vi "HW_Gantner_Refresh Tree Device Info.vi"(7 "Cfg":T1[](array[typedef]), 8 "error in":errorcluster caption="错误输入", 10 "Device":string="Device", 11 "Ref.Tree Ref":refnum<vi>) -> (0 "error out":errorcluster caption="错误输出")   [LabVIEW 2016]
uses:
  Ctrls/HardWare _ Module Configuration.ctl
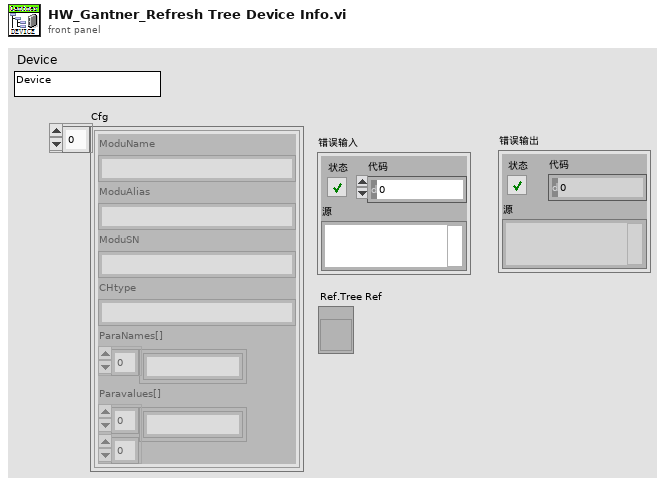
[diagram p1: front panel]
types:
  T1 = typedef "HardWare _ Module Configuration.ctl" = cluster{"ModuName":string, "ModuAlias":string, "ModuSN":string, "CHtype":string, "ParaNames[]":string[], "Paravalues[]":string[][]}
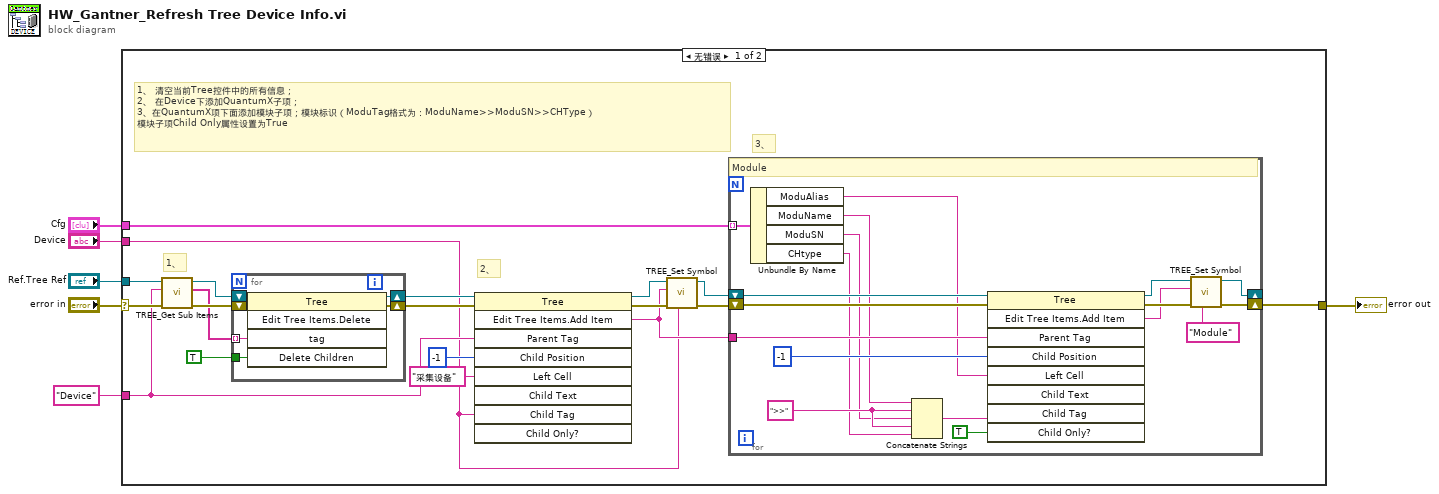
[diagram p0: block diagram]
diagram:
  n1 = case shown="无错误" "error in" {
    selector: "error in" -> [w21 w50]
    tunnel: [w25 w50] -> w5
    tunnel: "Ref.Tree Ref" -> [w19 _]
    tunnel: "Device" ("PicName") -> [w18 _]
    tunnel: "Cfg" -> [w9 _]
    tunnel: "Device" -> [w8 _]
    frame No Error {
      # "3、"
      # "2、"
      # "1、"
      # "1、 清空当前Tree控件中的所有信息；\n2、 在Device下添加QuantumX子项；\n3、在QuantumX项下面添加模块子项；模块标识（ModuTag格式为：ModuName>>ModuSN>>CHType）\n模块子项Child Only属性设置为True"
      n2 = call "TREE_Get Sub Items.vi"("error in"=w21, "Par Tag"=w18, "TreeRef"=w19) -> ("error out"=w20:errorcluster, "Tags"=w16:string[], "TreeRef"=w17:refnum<vi>)  [unwired: 5 in, 1 out]
      n3 = for {
        tunnel: TRUE ("删除子项？") -> [w47]
        shift-right: [w48] -> w23
        shift-left: w20 -> [w46]
        shift-right: [w49] -> w24
        shift-left: w17 -> [w45]
        tunnel: w16 -> [w44] mode=indexing
        n4 = invoke class="Tree" method="Edit Tree Items.Delete"(reference=w45, error in=w46, "tag"=w44, "Delete Children"=w47) -> (reference out=w49:refnum<vi>, error out=w48:errorcluster)  [unwired: 1 in, 3 out]
      }
      n5 = invoke class="Tree" method="Edit Tree Items.Add Item"(reference=w24, error in=w23, "Parent Tag"=w18, "Child Position"=-1 ("子项位置"), "Left Cell"="采集设备" ("左单元格字符串"), "Child Tag"=w8) -> (reference out=w13:refnum<vi>, error out=w15:errorcluster, "Edit Tree Items:Add Item"=w11:string)  [unwired: 3 in, 6 out]
      n6 = call "TREE_Set Symbol.vi"("PicName"=w8, "error in"=w15, "Tag"=w11, "Tree Ref"=w13) -> ("error out"=w14:errorcluster, "Tree Ref"=w12:refnum<vi>)  [unwired: 6 in]
      n7 = for {
        shift-right: [w34] -> _
        shift-left: w12 -> [w41]
        shift-right: [w36] -> w25
        shift-left: w14 -> [w40]
        tunnel: w11 -> [w38]
        tunnel: w9 -> [w43] mode=indexing
        w29 = ">>" ("字符串")
        # "Module"
        n8 = Unbundle By Name(w43) -> ("ModuAlias"=w27:string, "ModuName"=w30:string, "ModuSN"=w28:string, "CHtype"=w26:string)
        n9 = Concatenate Strings(w30, w29, w28, w29, w26) -> (w42:string)
        n10 = invoke class="Tree" method="Edit Tree Items.Add Item"(reference=w41, error in=w40, "Parent Tag"=w38, "Child Position"=-1 ("子项位置"), "Left Cell"=w27, "Child Tag"=w42, "Child Only?"=TRUE ("仅作为子项？")) -> (reference out=w35:refnum<vi>, error out=w37:errorcluster, "Edit Tree Items:Add Item"=w33:string)  [unwired: 2 in, 6 out]
        n11 = call "TREE_Set Symbol.vi"("PicName"="Module", "error in"=w37, "Tag"=w33, "Tree Ref"=w35) -> ("error out"=w36:errorcluster, "Tree Ref"=w34:refnum<vi>)  [unwired: 6 in]
      }
    }
    frame Error {
    }
  }
  "error out" <- w5
